vi "strObjectChoice.vi"(9 "ObjectChoice":i32[](listbox), 11 "btnSelectObject":bool) -> (1 "mu08ArrayIndexFinalOut":u8[](array[numeric]), 2 "NamePic":picture, 3 "mbfObjectChoiceArray":bool[](array[boolean]))   [LabVIEW 2011]
uses:
  <vilib>/Utility/miscctls.llb/LVPoint32TypeDef.ctl
panel:
  out "mbfStartDraw":bool
  out "btnSelectObject.Txt":string
  out "坐标":T1
  out "mu08ObjectArraySize":u8
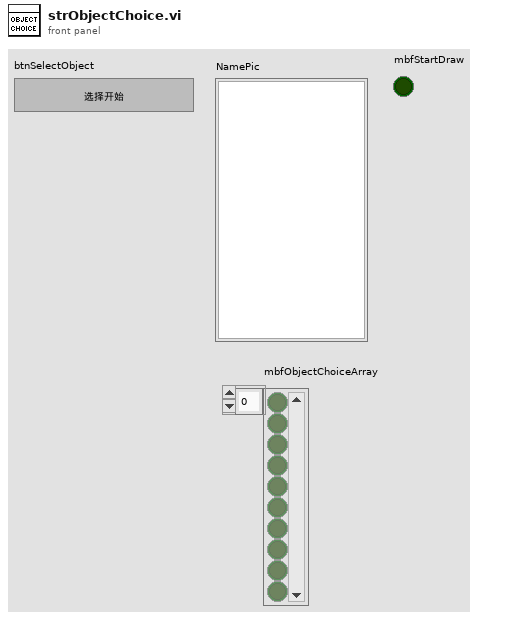
[diagram p1: front panel]
types:
  T1 = typedef "LVPoint32TypeDef.ctl" = cluster{"Horizontal":i32, "Vertical":i32}
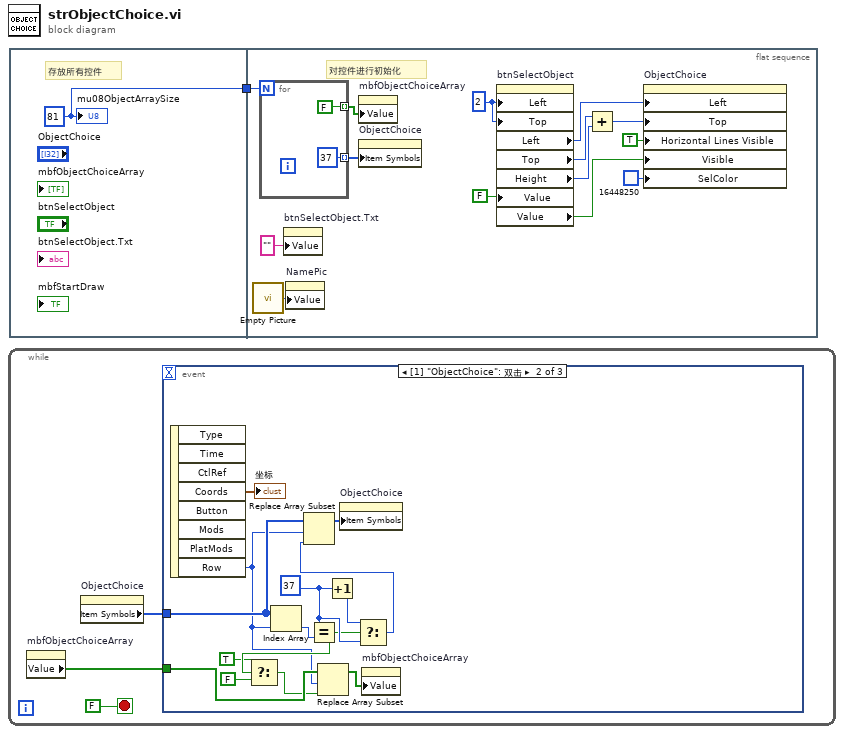
[diagram p0: block diagram]
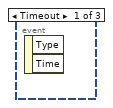
[diagram p2: hidden frame]
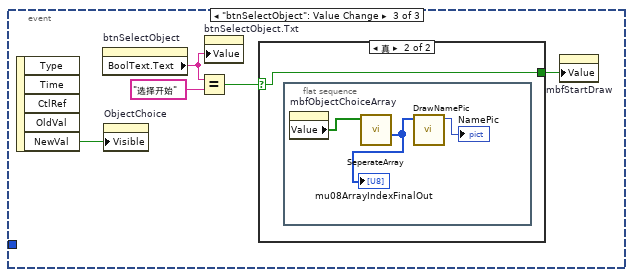
[diagram p3: hidden frame]
diagram:
  n1 = while {
    stop <- FALSE stop-if-true
    n2 = property on="mbfObjectChoiceArray" class="Arr (严格)"() -> ("Value"=w2:bool[])  [unwired: 2 in, 2 out]
    n3 = property on="ObjectChoice" class="LstBox (严格)"() -> ("Item Symbols"=w3:i32[])  [unwired: 2 in, 2 out]
    n4 = event shown="[1] \"ObjectChoice\": 双击" {
      selector: _ -> [_ _ _]
      dyn-events: _ -> [_ _ _]
      timeout: _ -> [_ _ _]
      tunnel: w3 -> [_ w17 _]
      tunnel: w2 -> [_ w8 _]
      event Timeout {
        n5 = event-data() -> ()  [unwired: 1 in, 2 out]
      }
      event "ObjectChoice": Double Click {
        w13 = 37 ("y")
        n6 = event-data() -> ("Coords"=→"坐标":T1, "Row"=w5:i32)  [unwired: 1 in, 6 out]
        n7 = Index Array(array=w17, index=w5) -> (element=w15:i32)
        n8 = Equal?(x=w13, y=w15) -> (x = y?=w11:bool)
        n9 = Select(t=TRUE, s=w11, f=FALSE) -> (s? t:f=w7:bool)
        n10 = Replace Array Subset(array=w8, new element=w7, index=w5) -> (w6:bool[])
        n11 = Increment(x=w13) -> (x+1=w14:i32)
        n12 = Select(t=w14, s=w11, f=w13) -> (s? t:f=w12:i32)
        n13 = Replace Array Subset(array=w17, new element=w12, index=w5) -> (w16:i32[])
        n14 = property on="ObjectChoice" class="LstBox (严格)"("Item Symbols"=w16) -> ()  [unwired: 2 in, 2 out]
        n15 = property on="mbfObjectChoiceArray" class="Arr (严格)"("Value"=w6) -> ()  [unwired: 2 in, 2 out]
      }
      event "btnSelectObject": Value Change {
        n16 = event-data() -> ("NewVal"=w23:bool)  [unwired: 1 in, 4 out]
        n17 = property on="btnSelectObject" class="Bool (严格)"() -> ("BoolText.Text"=w22:string)  [unwired: 2 in, 2 out]
        n18 = property on="ObjectChoice" class="LstBox (严格)"("Visible"=w23) -> ()  [unwired: 2 in, 2 out]
        n19 = Equal?(x=w22, y="选择开始") -> (x = y?=w20:bool)
        n20 = property on="btnSelectObject.Txt" class="Str"("Value"=w22) -> ()  [unwired: 2 in, 2 out]
        n21 = case shown="真" w20 {
          selector: w20 -> [w24 w25]
          tunnel: [w24 w25] -> w19
          frame False {
          }
          frame True {
            n22 = flat-sequence {
              frame #0 {
                n23 = property on="mbfObjectChoiceArray" class="Arr (严格)"() -> ("Value"=w28:bool[])  [unwired: 2 in, 2 out]
                n24 = call "SeperateArray.vi"("mbfArrayIn"=w28) -> ("mu08ArrayIndexFinalOut"=w27:u8[])  [unwired: 9 in, 1 out]
                "mu08ArrayIndexFinalOut" <- w27
                n25 = call "DrawNamePic.vi"("mu08ArrayIn"=w27) -> ("NamePic"=→"NamePic":picture)  [unwired: 10 in]
              }
            }
          }
        }
        n26 = property on="mbfStartDraw" class="Bool (严格)"("Value"=w19) -> ()  [unwired: 2 in, 2 out]
      }
    }
  }
  n27 = flat-sequence {
    tunnel: [w29] -> w1
    tunnel: w1 -> [w43]
    frame #0 {
      w29 = u8 81 ("mu08ObjectArraySize")
      # "存放所有控件"
      "mu08ObjectArraySize" <- w29
    }
    frame #1 {
      w35 = 2 ("位置:居左")
      # "对控件进行初始化"
      n28 = call "Empty Picture"() -> ("empty picture"=w30:picture)
      n29 = for {
        N: w43 -> [_]
        tunnel: [FALSE] -> w41 mode=indexing
        tunnel: [37] -> w42 mode=indexing
      }
      n30 = property on="btnSelectObject.Txt" class="Str"("Value"="" ("btnSelectObject.Txt")) -> ()  [unwired: 2 in, 2 out]
      n31 = property on="NamePic" class="Pict"("Value"=w30) -> ()  [unwired: 2 in, 2 out]
      n32 = property on="mbfObjectChoiceArray" class="Arr (严格)"("Value"=w41) -> ()  [unwired: 2 in, 2 out]
      n33 = property on="ObjectChoice" class="LstBox (严格)"("Item Symbols"=w42) -> ()  [unwired: 2 in, 2 out]
      n34 = property on="btnSelectObject" class="Bool (严格)"("Left"=w35, "Top"=w35, "Value"=FALSE ("btnSelectObject")) -> ("Left"=w40:i32, "Top"=w33:i32, "Height"=w39:u32, "Value"=w34:bool)  [unwired: 2 in, 2 out]
      n35 = Add(x=w33, y=w39) -> (x+y=w38:u32)
      n36 = property on="ObjectChoice" class="LstBox (严格)"("Left"=w40, "Top"=w38, "Horizontal Lines Visible"=TRUE, "Visible"=w34, "SelColor"=u32 16448250) -> ()  [unwired: 2 in, 2 out]
    }
  }
